vi "Move.vi"(1 "Enum":enum16{"forward", "backward", "left", "right"}(ring), 2 "distance":dbl, 3 "speed":i32) -> ()   [LabVIEW 2018]
uses:
  Comulative wheels angles.vi
panel:
  out "busy count":i32
  out "Numeric 4":i16
  out "Numeric 3":i16
  out "Numeric 2":i16
  out "Numeric":i16
  out "q":i32
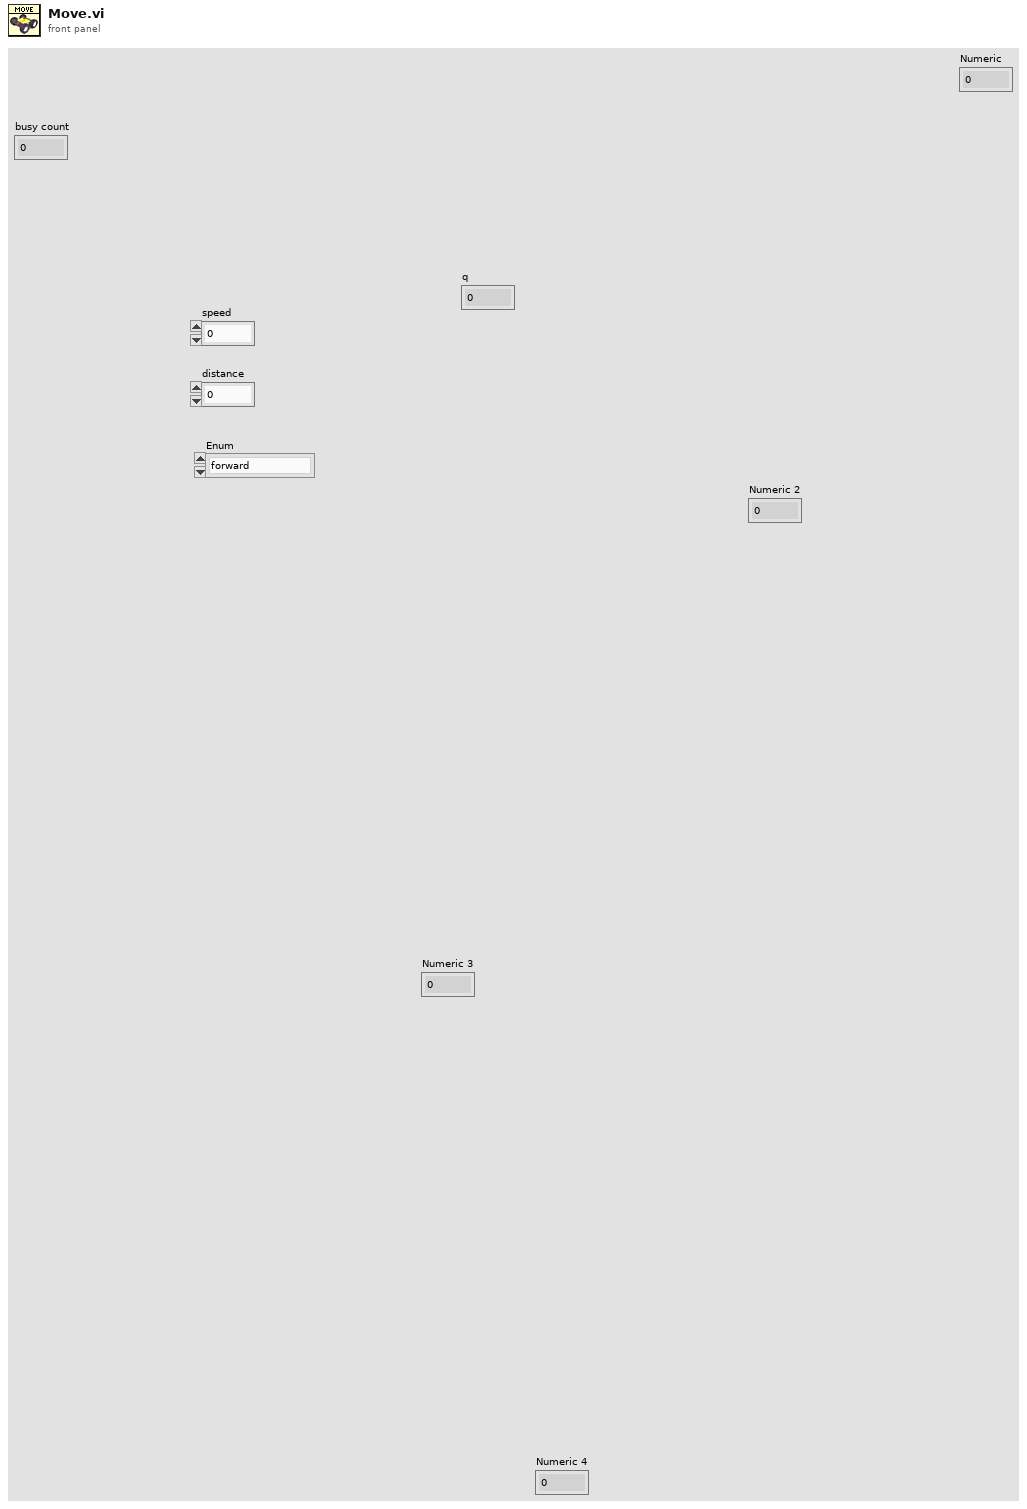
[diagram p1: front panel]
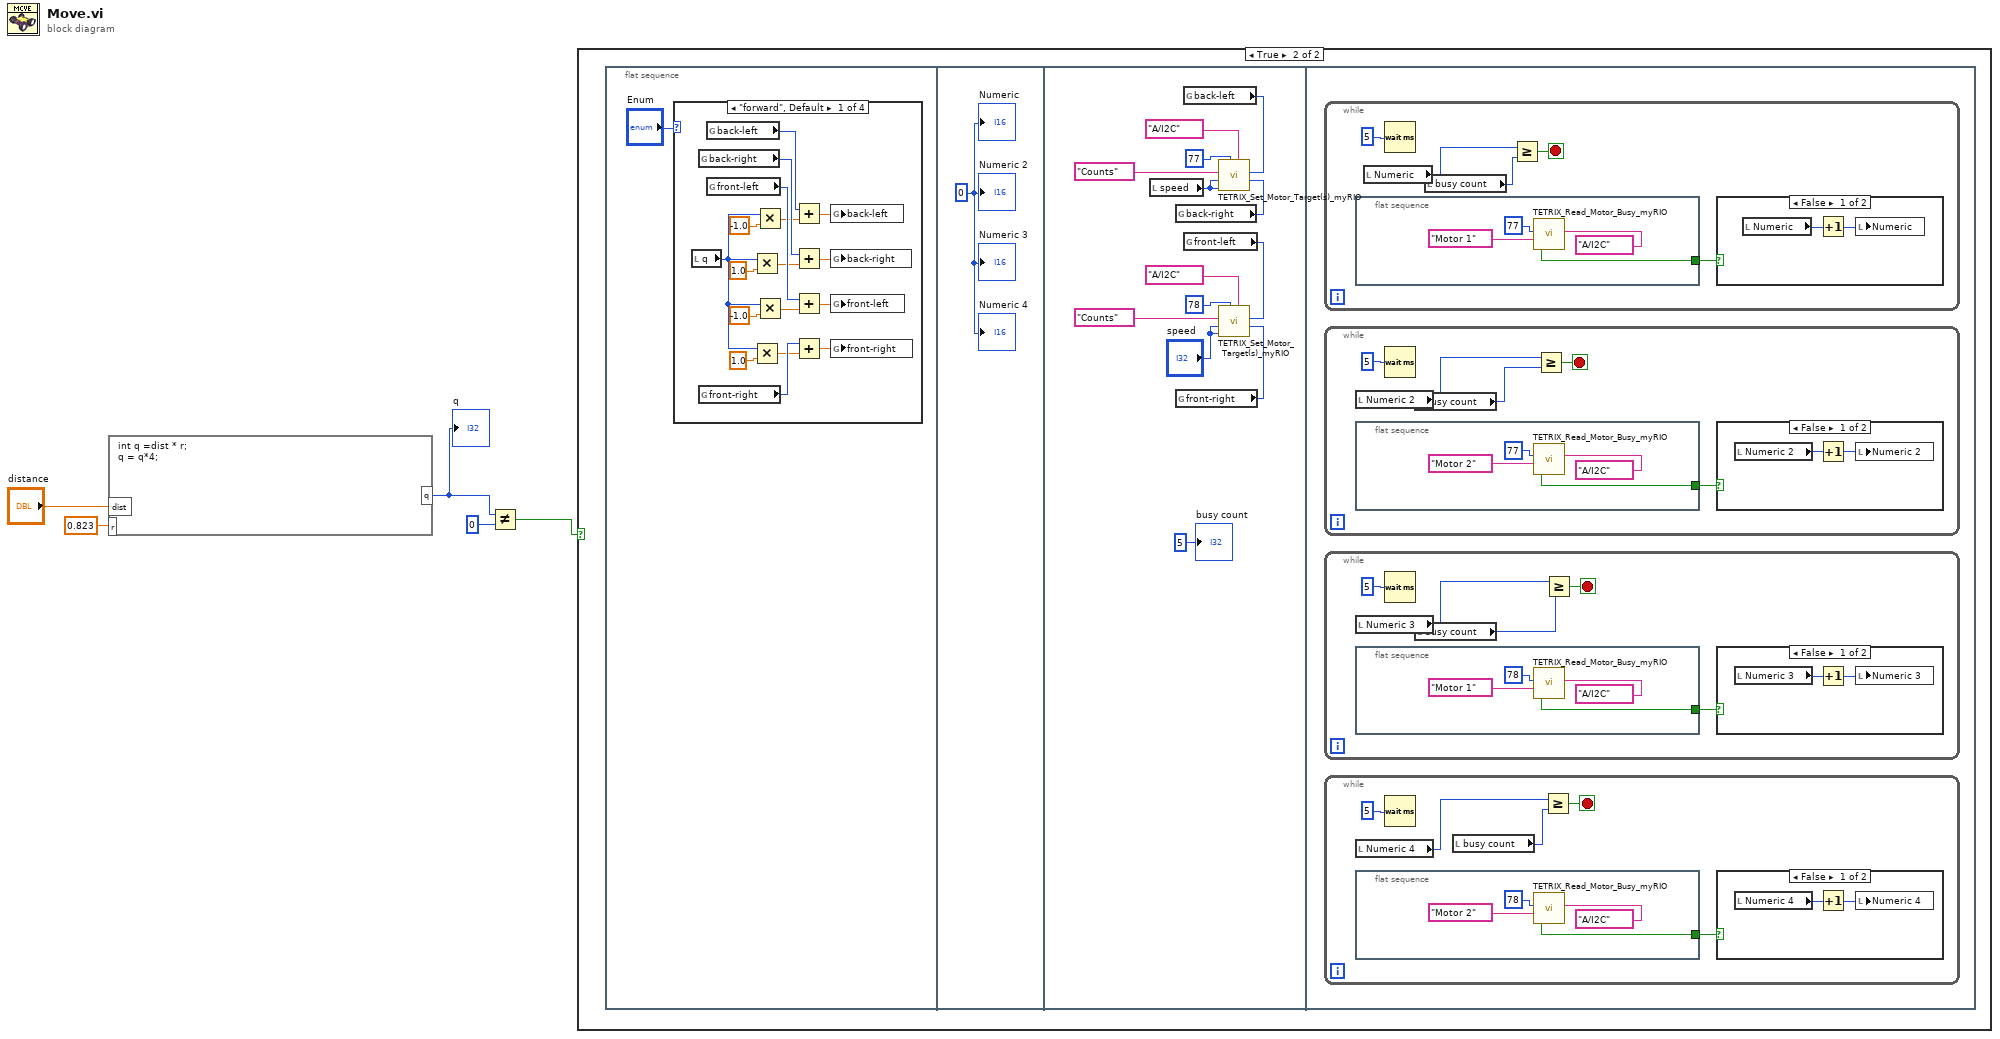
[diagram p0: block diagram]
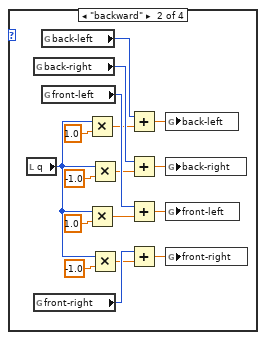
[diagram p3: hidden frame]
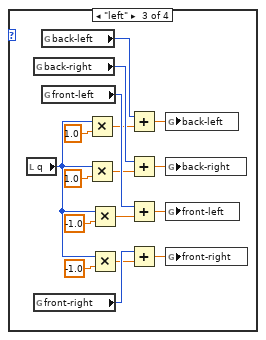
[diagram p4: hidden frame]
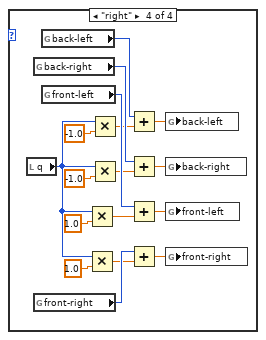
[diagram p5: hidden frame]
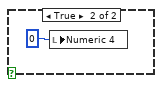
[diagram p6: hidden frame]
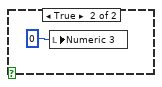
[diagram p7: hidden frame]
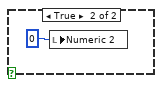
[diagram p8: hidden frame]
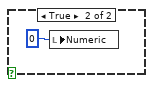
[diagram p9: hidden frame]
diagram:
  n1 = formula code="int q =dist * r;\nq = q*4;"("dist"="distance", "r"=0.823) -> ("q"=w3:i32)
  "q" <- w3
  n2 = Not Equal?(x=w3, y=0) -> (x != y?=w1:bool)
  n3 = case shown="True" w1 {
    frame False {
    }
    frame True {
      n4 = flat-sequence {
        frame #0 {
          n5 = case shown="\"forward\", Default" "Enum" {
            frame "forward", Default {
              n6 = local read "q"() -> (w7:i32)
              n7 = global read "Comulative wheels angles.vi" "back-right"() -> (w15:i32)
              n8 = global read "Comulative wheels angles.vi" "front-right"() -> (w23:i32)
              n9 = global read "Comulative wheels angles.vi" "back-left"() -> (w11:i32)
              n10 = global read "Comulative wheels angles.vi" "front-left"() -> (w19:i32)
              n11 = Multiply(x=w7, y=1.0) -> (x*y=w14:dbl)
              n12 = Multiply(x=w7, y=1.0) -> (x*y=w22:dbl)
              n13 = Multiply(x=w7, y=-1.0) -> (x*y=w10:dbl)
              n14 = Multiply(x=w7, y=-1.0) -> (x*y=w18:dbl)
              n15 = Add(x=w11, y=w10) -> (x+y=w8:dbl)
              n16 = Add(x=w15, y=w14) -> (x+y=w12:dbl)
              n17 = Add(x=w19, y=w18) -> (x+y=w16:dbl)
              n18 = Add(x=w23, y=w22) -> (x+y=w20:dbl)
              n19 = global write "Comulative wheels angles.vi" "back-left"(w8) -> ()
              n20 = global write "Comulative wheels angles.vi" "back-right"(w12) -> ()
              n21 = global write "Comulative wheels angles.vi" "front-left"(w16) -> ()
              n22 = global write "Comulative wheels angles.vi" "front-right"(w20) -> ()
            }
            frame "backward" {
              n23 = local read "q"() -> (w24:i32)
              n24 = global read "Comulative wheels angles.vi" "back-right"() -> (w32:i32)
              n25 = global read "Comulative wheels angles.vi" "front-right"() -> (w40:i32)
              n26 = global read "Comulative wheels angles.vi" "back-left"() -> (w28:i32)
              n27 = global read "Comulative wheels angles.vi" "front-left"() -> (w36:i32)
              n28 = Multiply(x=w24, y=1.0) -> (x*y=w27:dbl)
              n29 = Multiply(x=w24, y=1.0) -> (x*y=w35:dbl)
              n30 = Multiply(x=w24, y=-1.0) -> (x*y=w31:dbl)
              n31 = Multiply(x=w24, y=-1.0) -> (x*y=w39:dbl)
              n32 = Add(x=w28, y=w27) -> (x+y=w25:dbl)
              n33 = Add(x=w32, y=w31) -> (x+y=w29:dbl)
              n34 = Add(x=w36, y=w35) -> (x+y=w33:dbl)
              n35 = Add(x=w40, y=w39) -> (x+y=w37:dbl)
              n36 = global write "Comulative wheels angles.vi" "back-left"(w25) -> ()
              n37 = global write "Comulative wheels angles.vi" "back-right"(w29) -> ()
              n38 = global write "Comulative wheels angles.vi" "front-left"(w33) -> ()
              n39 = global write "Comulative wheels angles.vi" "front-right"(w37) -> ()
            }
            frame "left" {
              n40 = local read "q"() -> (w41:i32)
              n41 = global read "Comulative wheels angles.vi" "back-right"() -> (w49:i32)
              n42 = global read "Comulative wheels angles.vi" "front-right"() -> (w57:i32)
              n43 = global read "Comulative wheels angles.vi" "back-left"() -> (w45:i32)
              n44 = global read "Comulative wheels angles.vi" "front-left"() -> (w53:i32)
              n45 = Multiply(x=w41, y=1.0) -> (x*y=w44:dbl)
              n46 = Multiply(x=w41, y=1.0) -> (x*y=w48:dbl)
              n47 = Multiply(x=w41, y=-1.0) -> (x*y=w52:dbl)
              n48 = Multiply(x=w41, y=-1.0) -> (x*y=w56:dbl)
              n49 = Add(x=w45, y=w44) -> (x+y=w42:dbl)
              n50 = Add(x=w49, y=w48) -> (x+y=w46:dbl)
              n51 = Add(x=w53, y=w52) -> (x+y=w50:dbl)
              n52 = Add(x=w57, y=w56) -> (x+y=w54:dbl)
              n53 = global write "Comulative wheels angles.vi" "back-left"(w42) -> ()
              n54 = global write "Comulative wheels angles.vi" "back-right"(w46) -> ()
              n55 = global write "Comulative wheels angles.vi" "front-left"(w50) -> ()
              n56 = global write "Comulative wheels angles.vi" "front-right"(w54) -> ()
            }
            frame "right" {
              n57 = local read "q"() -> (w58:i32)
              n58 = global read "Comulative wheels angles.vi" "back-right"() -> (w66:i32)
              n59 = global read "Comulative wheels angles.vi" "front-right"() -> (w74:i32)
              n60 = global read "Comulative wheels angles.vi" "back-left"() -> (w62:i32)
              n61 = global read "Comulative wheels angles.vi" "front-left"() -> (w70:i32)
              n62 = Multiply(x=w58, y=1.0) -> (x*y=w69:dbl)
              n63 = Multiply(x=w58, y=1.0) -> (x*y=w73:dbl)
              n64 = Multiply(x=w58, y=-1.0) -> (x*y=w61:dbl)
              n65 = Multiply(x=w58, y=-1.0) -> (x*y=w65:dbl)
              n66 = Add(x=w62, y=w61) -> (x+y=w59:dbl)
              n67 = Add(x=w66, y=w65) -> (x+y=w63:dbl)
              n68 = Add(x=w70, y=w69) -> (x+y=w67:dbl)
              n69 = Add(x=w74, y=w73) -> (x+y=w71:dbl)
              n70 = global write "Comulative wheels angles.vi" "back-left"(w59) -> ()
              n71 = global write "Comulative wheels angles.vi" "back-right"(w63) -> ()
              n72 = global write "Comulative wheels angles.vi" "front-left"(w67) -> ()
              n73 = global write "Comulative wheels angles.vi" "front-right"(w71) -> ()
            }
          }
        }
        frame #1 {
          w75 = i16 0 ("Numeric")
          "Numeric" <- w75
          "Numeric 2" <- w75
          "Numeric 3" <- w75
          "Numeric 4" <- w75
        }
        frame #2 {
          n74 = local read "speed"() -> (w77:i32)
          n75 = global read "Comulative wheels angles.vi" "back-right"() -> (w79:i32)
          n76 = global read "Comulative wheels angles.vi" "front-right"() -> (w85:i32)
          n77 = global read "Comulative wheels angles.vi" "back-left"() -> (w80:i32)
          n78 = global read "Comulative wheels angles.vi" "front-left"() -> (w86:i32)
          n79 = call <vilib>:"TETRIX_Set_Motor_Target(s)_myRIO.vi"("Motor 2 Encoder Target"=w79, "Motor 1 Encoder Target"=w80, "myRIO MXP Port A/B"=tag "A/I2C", "Controller ID#  (I2C Address)"=u8 77, "Motor 2 Constant Speed (Degrees per Second)"=w77, "Motor 1 Contant Speed (Degrees per Second)"=w77, "Encoder Units"="Counts") -> ()  [unwired: 2 in, 1 out]
          n80 = call <vilib>:"TETRIX_Set_Motor_Target(s)_myRIO.vi"("Motor 2 Encoder Target"=w85, "Motor 1 Encoder Target"=w86, "myRIO MXP Port A/B"=tag "A/I2C", "Controller ID#  (I2C Address)"=u8 78, "Motor 2 Constant Speed (Degrees per Second)"="speed", "Motor 1 Contant Speed (Degrees per Second)"="speed", "Encoder Units"="Counts") -> ()  [unwired: 2 in, 1 out]
          "busy count" <- 5 ("busy count")
        }
        frame #3 {
          n81 = while {
            stop <- w127 stop-if-true
            n82 = flat-sequence {
              tunnel: [w133] -> w126
              frame #0 {
                n83 = call <vilib>:"TETRIX_Read_Motor_Busy_myRIO.vi"("myRIO MXP Port A/B"=tag "A/I2C", "Select Channel"="Motor 1", "Controller ID#  (I2C Address)"=u8 77) -> ("Motor Busy?"=w133:bool)  [unwired: 3 in, 1 out]
              }
            }
            n84 = local read "Numeric"() -> (w128:i16)
            n85 = Wait (ms)(milliseconds to wait=u32 5) -> ()  [unwired: 1 out]
            n86 = local read "busy count"() -> (w125:i32)
            n87 = Greater Or Equal?(x=w128, y=w125) -> (x >= y?=w127:bool)
            n88 = case shown="False" w126 {
              frame False {
                n89 = local read "Numeric"() -> (w131:i16)
                n90 = Increment(x=w131) -> (x+1=w130:i16)
                n91 = local write "Numeric"(w130) -> ()
              }
              frame True {
                n92 = local write "Numeric"(i16 0 ("Numeric")) -> ()
              }
            }
          }
          n93 = while {
            stop <- w115 stop-if-true
            n94 = local read "Numeric 2"() -> (w116:i16)
            n95 = flat-sequence {
              tunnel: [w122] -> w114
              frame #0 {
                n96 = call <vilib>:"TETRIX_Read_Motor_Busy_myRIO.vi"("myRIO MXP Port A/B"=tag "A/I2C", "Select Channel"="Motor 2", "Controller ID#  (I2C Address)"=u8 77) -> ("Motor Busy?"=w122:bool)  [unwired: 3 in, 1 out]
              }
            }
            n97 = Wait (ms)(milliseconds to wait=u32 5) -> ()  [unwired: 1 out]
            n98 = local read "busy count"() -> (w113:i32)
            n99 = Greater Or Equal?(x=w116, y=w113) -> (x >= y?=w115:bool)
            n100 = case shown="False" w114 {
              frame False {
                n101 = local read "Numeric 2"() -> (w119:i16)
                n102 = Increment(x=w119) -> (x+1=w118:i16)
                n103 = local write "Numeric 2"(w118) -> ()
              }
              frame True {
                n104 = local write "Numeric 2"(i16 0 ("Numeric")) -> ()
              }
            }
          }
          n105 = while {
            stop <- w103 stop-if-true
            n106 = local read "Numeric 3"() -> (w104:i16)
            n107 = flat-sequence {
              tunnel: [w109] -> w102
              frame #0 {
                n108 = call <vilib>:"TETRIX_Read_Motor_Busy_myRIO.vi"("myRIO MXP Port A/B"=tag "A/I2C", "Select Channel"="Motor 1", "Controller ID#  (I2C Address)"=u8 78) -> ("Motor Busy?"=w109:bool)  [unwired: 3 in, 1 out]
              }
            }
            n109 = Wait (ms)(milliseconds to wait=u32 5) -> ()  [unwired: 1 out]
            n110 = local read "busy count"() -> (w101:i32)
            n111 = Greater Or Equal?(x=w104, y=w101) -> (x >= y?=w103:bool)
            n112 = case shown="False" w102 {
              frame False {
                n113 = local read "Numeric 3"() -> (w107:i16)
                n114 = Increment(x=w107) -> (x+1=w106:i16)
                n115 = local write "Numeric 3"(w106) -> ()
              }
              frame True {
                n116 = local write "Numeric 3"(i16 0 ("Numeric")) -> ()
              }
            }
          }
          n117 = while {
            stop <- w91 stop-if-true
            n118 = local read "Numeric 4"() -> (w92:i16)
            n119 = flat-sequence {
              tunnel: [w97] -> w90
              frame #0 {
                n120 = call <vilib>:"TETRIX_Read_Motor_Busy_myRIO.vi"("myRIO MXP Port A/B"=tag "A/I2C", "Select Channel"="Motor 2", "Controller ID#  (I2C Address)"=u8 78) -> ("Motor Busy?"=w97:bool)  [unwired: 3 in, 1 out]
              }
            }
            n121 = Wait (ms)(milliseconds to wait=u32 5) -> ()  [unwired: 1 out]
            n122 = local read "busy count"() -> (w89:i32)
            n123 = Greater Or Equal?(x=w92, y=w89) -> (x >= y?=w91:bool)
            n124 = case shown="False" w90 {
              frame False {
                n125 = local read "Numeric 4"() -> (w95:i16)
                n126 = Increment(x=w95) -> (x+1=w94:i16)
                n127 = local write "Numeric 4"(w94) -> ()
              }
              frame True {
                n128 = local write "Numeric 4"(i16 0 ("Numeric")) -> ()
              }
            }
          }
        }
      }
    }
  }
